vi "Measurement renamer.vi"(4 "error in (no error)":errorcluster, 6 "Comment In":string, 7 "Measurement name In":string) -> (0 "error out":errorcluster, 1 "Canceled":bool, 2 "Comment Out":string, 3 "Measurement name Out":string)   [LabVIEW 2019]
doc: "Handles renaming of a measurement, displays a GUI window"
uses:
  <vilib>/Utility/miscctls.llb/LVPointTypeDef.ctl
panel:
  in  "Cancel":bool
  in  "Apply":bool
  in  "Comment":string
  in  "Measurment name":string
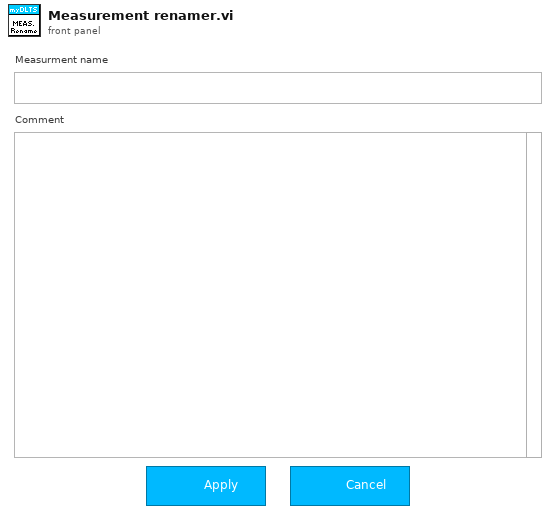
[diagram p1: front panel]
types:
  T1 = enum8{"Enabled", "Disabled", "Disabled and Grayed Out"}
  T2 = typedef "LVPointTypeDef.ctl" = cluster{"Horizontal":i16, "Vertical":i16}
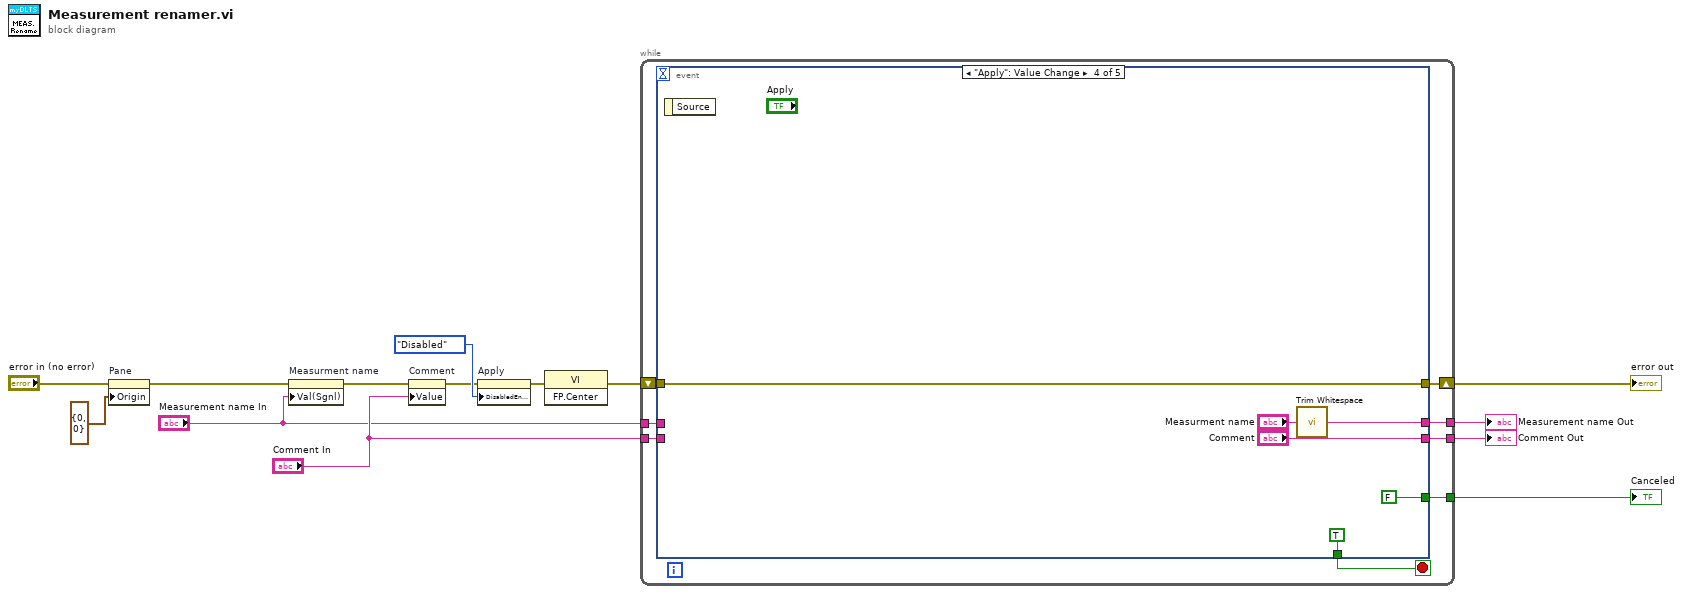
[diagram p0: block diagram]
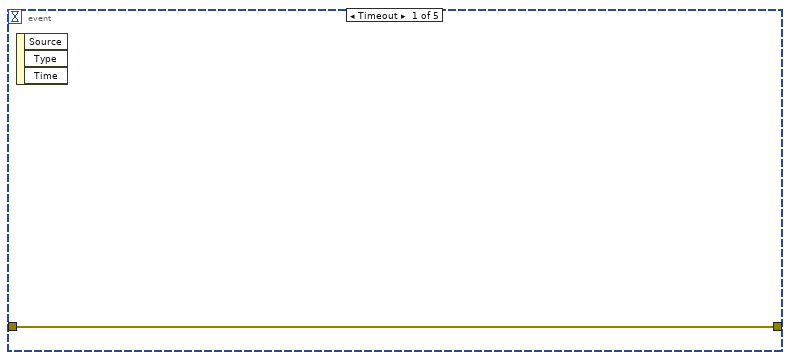
[diagram p2: hidden frame]
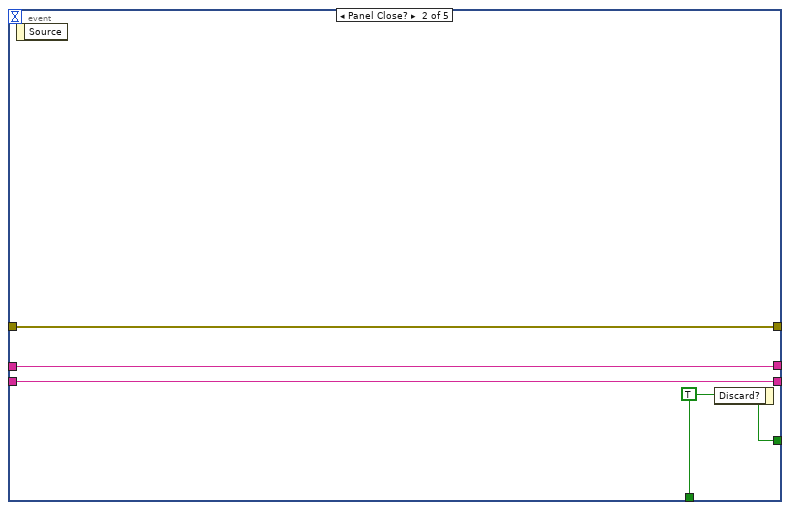
[diagram p3: hidden frame]
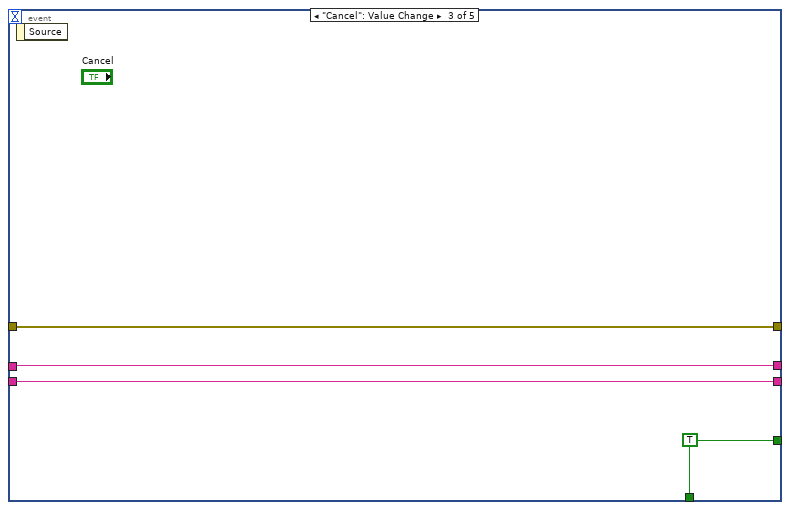
[diagram p4: hidden frame]
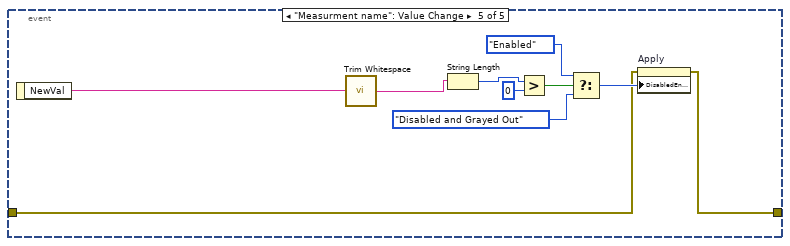
[diagram p5: hidden frame]
diagram:
  n1 = property on="Pane" class="Pane"(error in="error in (no error)", "Origin"=T2 {"Horizontal"=0, "Vertical"=0}) -> (error out=w13:errorcluster)  [unwired: 1 in, 1 out]
  n2 = property on="Measurment name" class="Str"(error in=w13, "Val(Sgnl)"="Measurement name In") -> (error out=w9:errorcluster)  [unwired: 1 in, 1 out]
  n3 = property on="Comment" class="Str"(error in=w9, "Value"="Comment In") -> (error out=w7:errorcluster)  [unwired: 1 in, 1 out]
  n4 = property on="Apply" class="Bool"(error in=w7, "DisabledEnum"=T1."Disabled" ("Disabled")) -> (error out=w6:errorcluster)  [unwired: 1 in, 1 out]
  n5 = invoke class="VI" method="FP.Center"(error in=w6) -> (error out=w5:errorcluster)  [unwired: 2 in, 2 out]
  n6 = while {
    tunnel: [w21] -> w14
    shift-right: [w19] -> w11
    shift-left: w5 -> [w20]
    tunnel: [w18] -> w4
    tunnel: [w17] -> w3
    tunnel: "Comment In" -> [w16]
    tunnel: "Measurement name In" -> [w15]
    stop <- w22 stop-if-true
    n7 = event shown="[3] \"Apply\": Value Change" {
      selector: _ -> [_ _ _ _ _]
      dyn-events: _ -> [_ _ _ _ _]
      timeout: _ -> [_ _ _ _ _]
      tunnel: [_ w27 w31 TRUE ("Discard?") _] -> w22
      tunnel: [_ w27 w31 FALSE ("Discard?") _] -> w21
      tunnel: w20 -> [w23 w26 w30 w34 w42]
      tunnel: [w23 w26 w30 w34 w43] -> w19
      tunnel: [_ w24 w29 w33 _] -> w18
      tunnel: [_ w25 w28 "Comment" _] -> w17
      tunnel: w16 -> [_ w25 w28 _ _]
      tunnel: w15 -> [_ w24 w29 _ _]
      event Timeout {
        n8 = event-data() -> ()  [unwired: 1 in, 3 out]
      }
      event Panel Close? {
        w27 = TRUE ("Discard?")
        n9 = event-data() -> ()  [unwired: 1 in, 1 out]
        n10 = event-data("Discard?"=w27) -> ()  [unwired: 1 in, 1 out]
      }
      event "Cancel": Value Change {
        w31 = TRUE ("Discard?")
        n11 = event-data() -> ()  [unwired: 1 in, 1 out]
      }
      event "Apply": Value Change {
        n12 = event-data() -> ()  [unwired: 1 in, 1 out]
        n13 = call <vilib>:"Trim Whitespace.vi"("string"="Measurment name") -> ("trimmed string"=w33:string)  [unwired: 1 in]
      }
      event "Measurment name": Value Change {
        n14 = event-data() -> ("NewVal"=w45:string)  [unwired: 1 in]
        n15 = call <vilib>:"Trim Whitespace.vi"("string"=w45) -> ("trimmed string"=w41:string)  [unwired: 1 in]
        n16 = String Length(string=w41) -> (length=w39:i32)
        n17 = Greater?(x=w39, y=0) -> (0:w38:bool)
        n18 = Select(t=T1."Enabled" ("Disabled"), s=w38, f=T1."Disabled and Grayed Out") -> (s? t:f=w44:T1)
        n19 = property on="Apply" class="Bool"(error in=w42, "DisabledEnum"=w44) -> (error out=w43:errorcluster)  [unwired: 1 in, 1 out]
      }
    }
  }
  "Canceled" <- w14
  "error out" <- w11
  "Comment Out" <- w3
  "Measurement name Out" <- w4
